vi "Magnet constants FGV.vi"(3 "Action":T2, 5 "Magnet Constants in":T1={"Switch resistant [K]"=5.0, "Switch superconducting [K]"=4.0, "First stage critical temperature [K]"=50.0, "Second stage critical temperature [K]"=5.0, "Inner magnet critical temperature [K]"=6.0, "Outer magnet critical temperature [K]"=5.0, "Field Constant [T/A]"=0.14911, "Maximum Current [A]"=107.3, "Maximum field [T]"=16.0, "Maximum source ramp [A/s]"=0.5, "Source precision [T]"=2e-05, "Ramp limits [A/s]"=[0.0506, 0.038, 0.0285, 0.0213, 0.0104], "Field limits [T]"=[3.0, 9.6, 13.3, 15.5, 16.0], "SMS"="COM3", "LSC218"="COM1"}) -> (2 "Magnet Constants out":T1={"Switch resistant [K]"=5.0, "Switch superconducting [K]"=4.0, "First stage critical temperature [K]"=50.0, "Second stage critical temperature [K]"=5.0, "Inner magnet critical temperature [K]"=6.0, "Outer magnet critical temperature [K]"=5.0, "Field Constant [T/A]"=0.14911, "Maximum Current [A]"=107.3, "Maximum field [T]"=16.0, "Maximum source ramp [A/s]"=0.5, "Source precision [T]"=2e-05, "Ramp limits [A/s]"=[0.0506, 0.038, 0.0285, 0.0213, 0.0104], "Field limits [T]"=[3.0, 9.6, 13.3, 15.5, 16.0], "SMS"="COM3", "LSC218"="COM1"})   [LabVIEW 2017, in "Magnet module.lvlib"]
uses:
  ctl/FGV action.ctl
  ctl/Magnet config constants.ctl
  Magnet module.lvlib
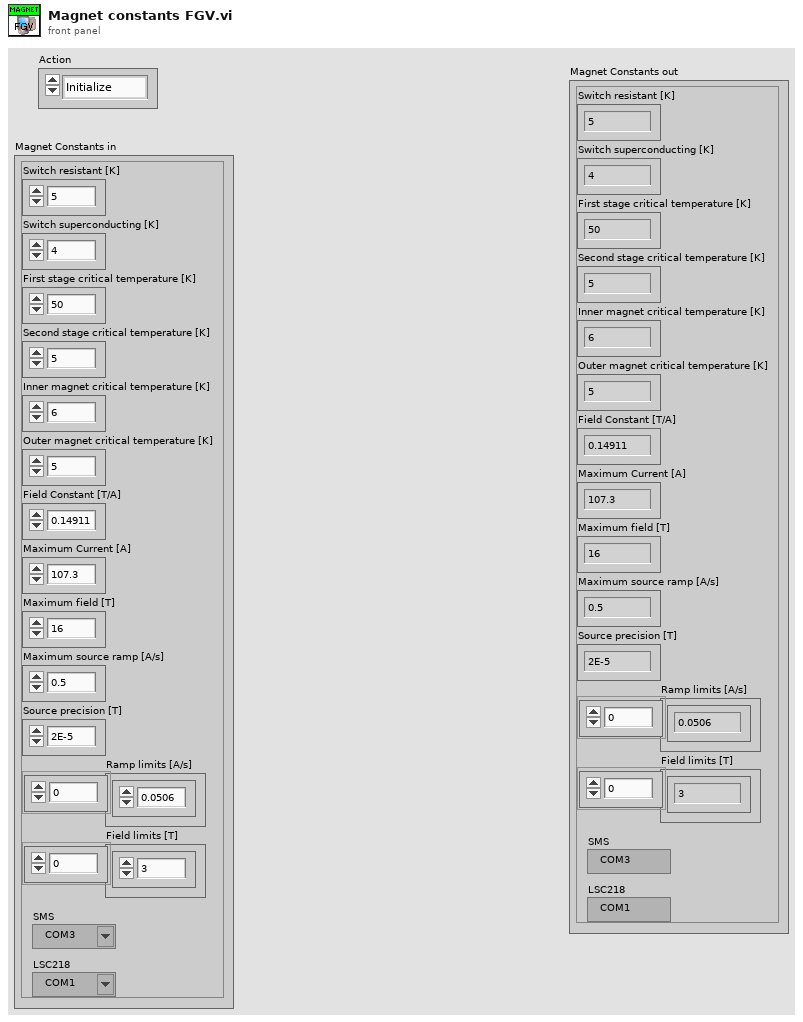
[diagram p1: front panel]
types:
  T1 = typedef "Magnet module.lvlib/Magnet config constants.ctl" = cluster{"Switch resistant [K]":dbl, "Switch superconducting [K]":dbl, "First stage critical temperature [K]":dbl, "Second stage critical temperature [K]":dbl, "Inner magnet critical temperature [K]":dbl, "Outer magnet critical temperature [K]":dbl, "Field Constant [T/A]":dbl, "Maximum Current [A]":dbl, "Maximum field [T]":dbl, "Maximum source ramp [A/s]":dbl, "Source precision [T]":dbl, "Ramp limits [A/s]":dbl[], "Field limits [T]":dbl[], "SMS":refnum<visa-resource-name>, "LSC218":refnum<visa-resource-name>}
  T2 = typedef "Magnet module.lvlib/FGV action.ctl" = enum16{"Initialize", "Update", "Read", "Action"}
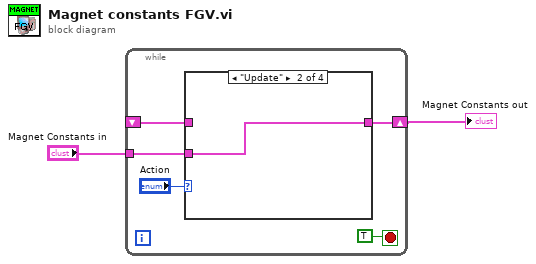
[diagram p0: block diagram]
diagram:
  n1 = while {
    shift-right: [w4] -> w1
    shift-left: _ -> [w5]
    tunnel: "Magnet Constants in" -> [w3]
    stop <- TRUE stop-if-true
    n2 = case shown="\"Update\"" "Action" {
      tunnel: w5 -> [_ _ w10 w11]
      tunnel: [w8 w9 w10 w11] -> w4
      tunnel: w3 -> [w8 w9 _ _]
      frame "Initialize", Default {
      }
      frame "Update" {
      }
      frame "Read" {
      }
      frame "Action" {
      }
    }
  }
  "Magnet Constants out" <- w1
